vi "checkfinishstep2.vi"(10 "Index":i32, 11 "StepNumber":i32[](array[numeric])=[0, -1, 1, -1, -1, 8, -1, -1, 3, -1, 4, -1, 5, 6, 7, 2, 9, 10]) -> (1 "ok":bool, 2 "Index":i32, 3 "Step":i32)   [LabVIEW 2019]
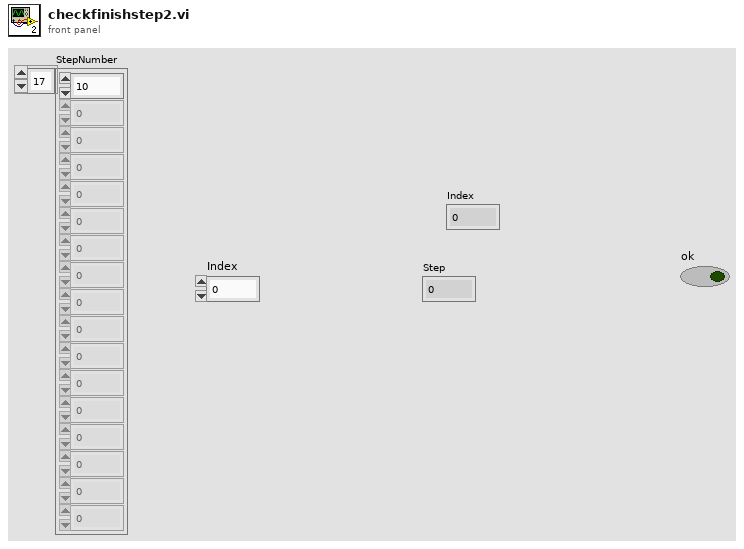
[diagram p1: front panel]
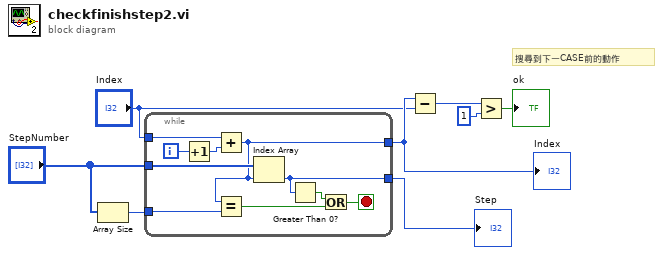
[diagram p0: block diagram]
diagram:
  # "搜尋到下一CASE前的動作"
  n1 = Array Size(array="StepNumber") -> (size(s)=w1:i32)
  n2 = while {
    tunnel: "StepNumber" -> [w18]
    tunnel: "Index" -> [w15]
    tunnel: [w16] -> w7
    tunnel: [w9] -> w6
    tunnel: w1 -> [w14]
    i -> [w17]
    stop <- w11 stop-if-true
    n3 = Increment(x=w17) -> (x+1=w10:i32)
    n4 = Add(x=w15, y=w10) -> (x+y=w9:i32)
    n5 = Equal?(x=w9, y=w14) -> (x = y?=w12:bool)
    n6 = Index Array(array=w18, index=w9) -> (element=w16:i32)
    n7 = Greater Than 0?(x=w16) -> (x > 0?=w13:bool)
    n8 = Or(x=w13, y=w12) -> (x .or. y?=w11:bool)
  }
  "Step" <- w7
  "Index" <- w6
  n9 = Subtract(x=w6, y="Index") -> (x-y=w4:i32)
  n10 = Greater?(x=w4, y=1) -> (0:→"ok":bool)
